vi "Direttore.fpga.vi"   [LabVIEW 2012]
uses:
  <vilib>/rvi/interface/RandomDataEmulation/nirviRandomDataFPGAFIFO.vi
  <vilib>/rvi/interface/RandomDataEmulation/niFpgaRandomDataHandleErrors.vi
  <vilib>/rvi/DataTransferAndStorage/Container/Common/niFpgaContainerGetUniqueNameForEmu.vi
  <vilib>/rvi/Memory/Memory_Emulation/niFpgaMemoryEmulationCacheClearOnFirstRun.vi
  <vilib>/rvi/Memory/Memory_Emulation/nirvimemoryEmulationManagerCache_MakeExclusive.vi
  <vilib>/rvi/Memory/Memory_Emulation/niFpgaMemoryEmulationValidateCache.vi
  <vilib>/rvi/Memory/Memory_Emulation/nirvimemoryEmulationManagerCache_ReleaseExclusive.vi
  <vilib>/rvi/Memory/Memory_Emulation/nirvimemoryEmulationManagerCache_InsertValue.vi
  <vilib>/Utility/error.llb/Clear Errors.vi
  <vilib>/rvi/Emulation/niFpgaSctlEmulationGetInTimedLoop.vi
  <vilib>/rvi/Memory/Memory_Emulation/nirvimemoryEmulationManagerCache_GetValue.vi
  <vilib>/rvi/Memory/Memory_Emulation/nirvimemoryEmulationManagerCache_SetValue.vi
  <vilib>/rvi/Emulation/niFpgaSctlEmulationResourceMgr.vi
  <vilib>/rvi/DataTransferAndStorage/Container/XNode/niFpgaContainer.xnode
  <vilib>/rvi/interface/RandomDataEmulation/nirviRandomDataFpgaReadWriteTemplate.vi
  <vilib>/rvi/Memory/Memory_Emulation/nirvimemoryEmulation.vi
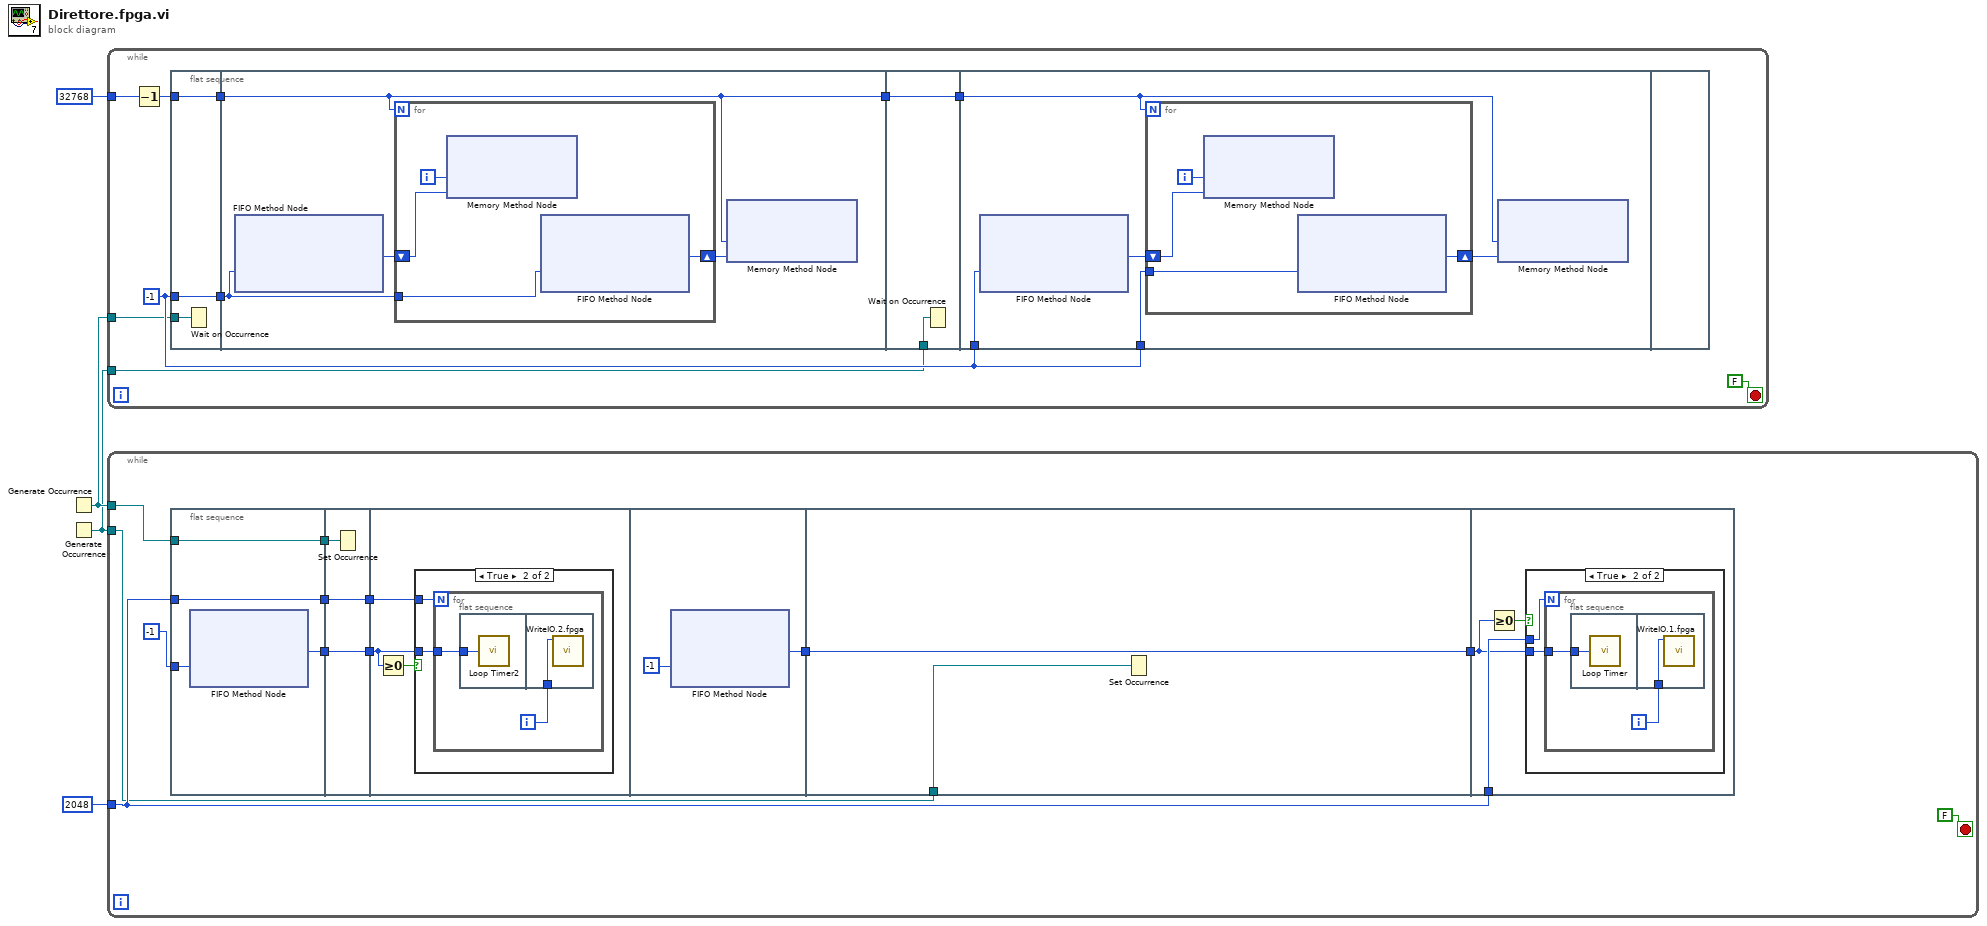
[diagram p0: block diagram]
diagram:
  n1 = Generate Occurrence() -> (w2:refnum<k4>)
  n2 = Generate Occurrence() -> (w1:refnum<k4>)
  n3 = while {
    tunnel: 32768 ("Numeric") -> [w14]
    tunnel: w2 -> [w7]
    tunnel: w1 -> [w6]
    stop <- FALSE stop-if-true
    w12 = -1 ("Timeout")
    n4 = Decrement(x=w14) -> (x-1=w13:i32)
    n5 = flat-sequence {
      tunnel: w12 -> [w16]
      tunnel: w13 -> [w17]
      tunnel: [w17] -> w9
      tunnel: [w16] -> w8
      tunnel: w7 -> [w15]
      tunnel: [w18] -> w11
      tunnel: w9 -> [w18]
      tunnel: w8 -> [w19]
      tunnel: w11 -> [w27]
      tunnel: [w27] -> w10
      tunnel: w6 -> [w26]
      tunnel: w10 -> [w28]
      tunnel: w12 -> [w30]
      tunnel: w12 -> [w29]
      frame #0 {
        n6 = Wait on Occurrence(2:w15) -> ()  [unwired: 2 in, 1 out]
      }
      frame #1 {
        n7 = xnode ("FIFO Method Node")("Timeout"=w19) -> ("Element"=w21:i16)  [unwired: 1 in, 2 out]
        n8 = for {
          N: w18 -> [_]
          shift-right: [w24] -> w20
          shift-left: w21 -> [w25]
          tunnel: w19 -> [w22]
          i -> [w23]
          n9 = xnode ("Memory Method Node")("Address"=w23, "Data"=w25) -> ()  [unwired: 1 in, 1 out]
          n10 = xnode ("FIFO Method Node")("Timeout"=w22) -> ("Element"=w24:i16)  [unwired: 1 in, 2 out]
        }
        n11 = xnode ("Memory Method Node")("Address"=w18, "Data"=w20) -> ()  [unwired: 1 in, 1 out]
      }
      frame #2 {
        n12 = Wait on Occurrence(2:w26) -> ()  [unwired: 2 in, 1 out]
      }
      frame #3 {
        n13 = xnode ("FIFO Method Node")("Timeout"=w29) -> ("Element"=w32:i16)  [unwired: 1 in, 2 out]
        n14 = for {
          N: w28 -> [_]
          shift-right: [w35] -> w31
          shift-left: w32 -> [w36]
          tunnel: w30 -> [w33]
          i -> [w34]
          n15 = xnode ("Memory Method Node")("Address"=w34, "Data"=w36) -> ()  [unwired: 1 in, 1 out]
          n16 = xnode ("FIFO Method Node")("Timeout"=w33) -> ("Element"=w35:i16)  [unwired: 1 in, 2 out]
        }
        n17 = xnode ("Memory Method Node")("Address"=w28, "Data"=w31) -> ()  [unwired: 1 in, 1 out]
      }
      frame #4 {
      }
    }
  }
  n18 = while {
    tunnel: u32 2048 -> [w48]
    tunnel: w2 -> [w46]
    tunnel: w1 -> [w38]
    stop <- FALSE stop-if-true
    n19 = flat-sequence {
      tunnel: [w52] -> w45
      tunnel: [w51] -> w43
      tunnel: [w49] -> w41
      tunnel: w48 -> [w52]
      tunnel: -1 ("Timeout") -> [w50]
      tunnel: w46 -> [w49]
      tunnel: w45 -> [w55]
      tunnel: [w55] -> w44
      tunnel: w43 -> [w54]
      tunnel: [w54] -> w42
      tunnel: w41 -> [w53]
      tunnel: w44 -> [w58]
      tunnel: w42 -> [w57]
      tunnel: [w65] -> w40
      tunnel: w40 -> [w68]
      tunnel: [w68] -> w39
      tunnel: w38 -> [w67]
      tunnel: w39 -> [w69]
      tunnel: w48 -> [w71]
      frame #0 {
        n20 = xnode ("FIFO Method Node")("Timeout"=w50) -> ("Element"=w51:i16)  [unwired: 1 in, 2 out]
      }
      frame #1 {
        n21 = Set Occurrence(w53) -> ()
      }
      frame #2 {
        n22 = Greater Or Equal To 0?(x=w57) -> (x >= 0?=w56:bool)
        n23 = case shown="True" w56 {
          tunnel: w58 -> [_ w60]
          tunnel: w57 -> [_ w59]
          frame False {
          }
          frame True {
            n24 = for {
              N: w60 -> [_]
              tunnel: w59 -> [w61]
              i -> [w62]
              n25 = flat-sequence {
                tunnel: w61 -> [w63]
                tunnel: w62 -> [w64]
                frame #0 {
                  n26 = call "Loop Timer2"("Count(uSec)"=w63) -> ()  [unwired: 1 out]
                }
                frame #1 {
                  n27 = call "WriteIO.2.fpga.vi"("x"=w64) -> ()  [unwired: 11 in]
                }
              }
            }
          }
        }
      }
      frame #3 {
        n28 = xnode ("FIFO Method Node")("Timeout"=-1) -> ("Element"=w65:i16)  [unwired: 1 in, 2 out]
      }
      frame #4 {
        n29 = Set Occurrence(w67) -> ()
      }
      frame #5 {
        n30 = Greater Or Equal To 0?(x=w69) -> (x >= 0?=w70:bool)
        n31 = case shown="True" w70 {
          tunnel: w69 -> [_ w73]
          tunnel: w71 -> [_ w72]
          frame False {
          }
          frame True {
            n32 = for {
              N: w72 -> [_]
              tunnel: w73 -> [w74]
              i -> [w75]
              n33 = flat-sequence {
                tunnel: w74 -> [w76]
                tunnel: w75 -> [w77]
                frame #0 {
                  n34 = call "Loop Timer"("Count(uSec)"=w76) -> ()  [unwired: 1 out]
                }
                frame #1 {
                  n35 = call "WriteIO.1.fpga.vi"("x"=w77) -> ()  [unwired: 11 in]
                }
              }
            }
          }
        }
      }
    }
  }
